vi "Create Cursor Plane.vi"(4 "Actual Range":T2, 5 "Cursor Plane":T3, 7 "Cursor Position":T1, 8 "error in (no error)":errorcluster, 11 "Cursor Object In":refnum<vi>) -> (0 "error out":errorcluster, 3 "Cursor Object Out":refnum<vi>)   [LabVIEW 2017, in "3D Plot.lvclass"]
uses:
  <vilib>/Math Plots/3D Math Plots/3D Plot/3D Plot/3D Plot.lvclass
  <vilib>/Math Plots/3D Math Plots/3D Plot/3D Plot/Typedef/Cursor Plane.ctl
  <vilib>/Math Plots/3D Math Plots/3D Plot/3D Plot/Typedef/Range Clusters.ctl
  <vilib>/picture/3D Picture Control/NI_3D Picture Control.lvlib
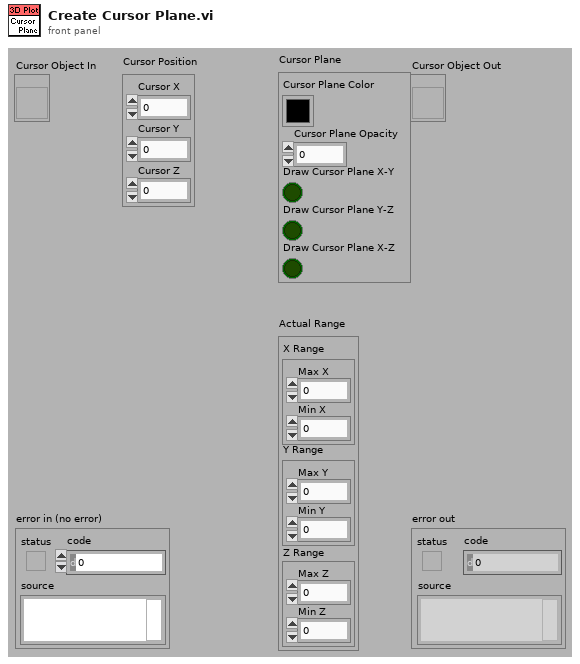
[diagram p1: front panel]
types:
  T1 = cluster{"Cursor X":sgl, "Cursor Y":sgl, "Cursor Z":sgl}
  T2 = typedef "3D Plot.lvclass/Range Clusters.ctl" = cluster{"X Range":cluster{"Max X":sgl, "Min X":sgl}, "Y Range":cluster{"Max Y":sgl, "Min Y":sgl}, "Z Range":cluster{"Max Z":sgl, "Min Z":sgl}}
  T3 = typedef "3D Plot.lvclass/Cursor Plane.ctl" = cluster{"Cursor Plane Color":u32, "Cursor Plane Opacity":sgl, "Draw Cursor Plane X-Z":bool, "Draw Cursor Plane Y-Z":bool, "Draw Cursor Plane X-Y":bool}
  T4 = enum16{"Normal Bin", "Opaque Bin", "Transparent Bin"}
  T5 = enum16{"Inherit Material", "Use entire Material", "Ignore Ambient", "Ignore Diffuse", "Ignore Specular", "Ignore Emission", "Ignore Ambient and Diffuse"}
  T6 = cluster{"X Range":cluster{"Max X":sgl, "Min X":sgl}, "Y Range":cluster{"Max Y":sgl, "Min Y":sgl}}
  T7 = cluster{"X Range":cluster{"Max X":sgl, "Min X":sgl}, "Z Range":cluster{"Max Z":sgl, "Min Z":sgl}}
  T8 = cluster{"Y Range":cluster{"Max Y":sgl, "Min Y":sgl}, "Z Range":cluster{"Max Z":sgl, "Min Z":sgl}}
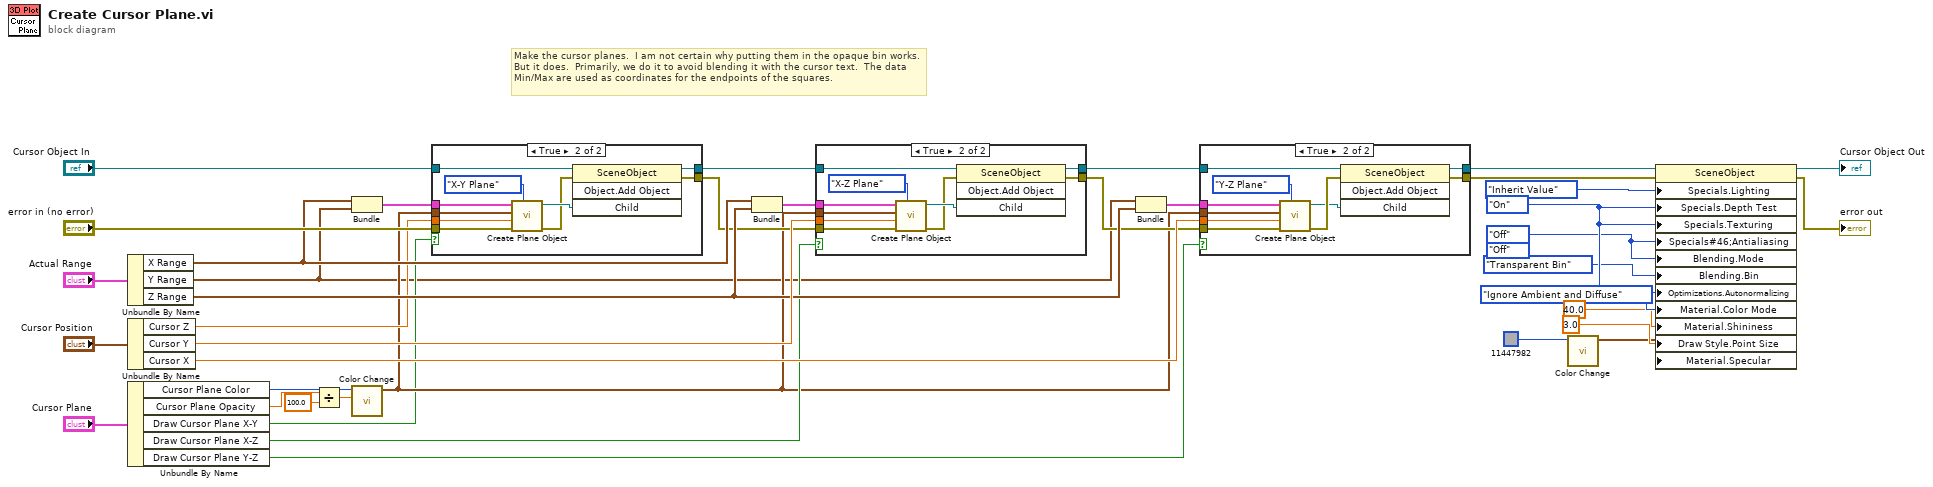
[diagram p0: block diagram]
diagram:
  (unwired) enum16{"Inherit Value", "Off", "On"}."Off" ("Blending:Mode")
  w6 = enum16{"Inherit Value", "Off", "On"}."On" ("Specials:Depth Test")
  w1 = enum16{"Inherit Value", "Off", "On"}."Off" ("Specials:Antialiasing")
  # "Make the cursor planes.  I am not certain why putting them in the opaque bin works.  But it does.  Primarily, we do it to avoid blending it with the cursor text.  The data Min/Max are used as coordinates for the endpoints of the squares."
  n1 = Unbundle By Name("Actual Range") -> ("X Range"=w27:cluster{"Max X":sgl, "Min X":sgl}, "Y Range"=w13:cluster{"Max Y":sgl, "Min Y":sgl}, "Z Range"=w26:cluster{"Max Z":sgl, "Min Z":sgl})
  n2 = Unbundle By Name("Cursor Position") -> ("Cursor Z"=w23:sgl, "Cursor Y"=w28:sgl, "Cursor X"=w24:sgl)
  n3 = Unbundle By Name("Cursor Plane") -> ("Cursor Plane Color"=w32:u32, "Cursor Plane Opacity"=w2:sgl, "Draw Cursor Plane X-Y"=w15:bool, "Draw Cursor Plane X-Z"=w22:bool, "Draw Cursor Plane Y-Z"=w21:bool)
  n4 = Divide(x=w2, y=sgl 100.0) -> (x/y=w17:sgl)
  n5 = Bundle("X Range"=w27, "Y Range"=w13) -> (w31:T6)  [unwired: 1 out]
  n6 = call <vilib>:"Color Change.vi"("Alpha"=w17, "Color"=w32) -> ("RGBA"=w16:cluster{"R":sgl, "G":sgl, "B":sgl, "A":sgl})  [unwired: 9 out]
  n7 = case shown="True" w15 {
    tunnel: w23 -> [_ w47]
    tunnel: w31 -> [_ w48]
    tunnel: w16 -> [_ w43]
    tunnel: "Cursor Object In" -> [w41 w51]
    tunnel: [w41 w49] -> w30
    tunnel: "error in (no error)" -> [w40 w46]
    tunnel: [w40 w50] -> w20
    frame False {
    }
    frame True {
      n8 = call <vilib>:"Create Plane Object.vi"("Plane"=enum16{"X-Y Plane", "Y-Z Plane", "X-Z Plane"}."X-Y Plane", "error in (no error)"=w46, "Offset"=w47, "RGBA"=w43, "Range Cluster"=w48) -> ("error out"=w44:errorcluster, "Cursor Plane Object"=w45:refnum<vi>)  [unwired: 1 in, 4 out]
      n9 = invoke class="SceneObject" method="Object.Add Object"(reference=w51, error in=w44, "Child"=w45) -> (reference out=w49:refnum<vi>, error out=w50:errorcluster)  [unwired: 1 in, 2 out]
    }
  }
  n10 = Bundle("X Range"=w27, "Z Range"=w26) -> (w14:T7)  [unwired: 1 out]
  n11 = case shown="True" w22 {
    tunnel: w28 -> [_ w60]
    tunnel: w14 -> [_ w59]
    tunnel: w16 -> [_ w55]
    tunnel: w30 -> [w53 w63]
    tunnel: [w53 w62] -> w29
    tunnel: w20 -> [w52 w56]
    tunnel: [w52 w61] -> w19
    frame False {
    }
    frame True {
      n12 = call <vilib>:"Create Plane Object.vi"("Plane"=enum16{"X-Y Plane", "Y-Z Plane", "X-Z Plane"}."X-Z Plane", "error in (no error)"=w56, "Offset"=w60, "RGBA"=w55, "Range Cluster"=w59) -> ("error out"=w57:errorcluster, "Cursor Plane Object"=w58:refnum<vi>)  [unwired: 1 in, 4 out]
      n13 = invoke class="SceneObject" method="Object.Add Object"(reference=w63, error in=w57, "Child"=w58) -> (reference out=w62:refnum<vi>, error out=w61:errorcluster)  [unwired: 1 in, 2 out]
    }
  }
  n14 = Bundle("Y Range"=w13, "Z Range"=w26) -> (w25:T8)  [unwired: 1 out]
  n15 = case shown="True" w21 {
    tunnel: w24 -> [_ w71]
    tunnel: w25 -> [_ w72]
    tunnel: w16 -> [_ w66]
    tunnel: w29 -> [w65 w75]
    tunnel: [w65 w74] -> w5
    tunnel: w19 -> [w64 w70]
    tunnel: [w64 w73] -> w4
    frame False {
    }
    frame True {
      n16 = call <vilib>:"Create Plane Object.vi"("Plane"=enum16{"X-Y Plane", "Y-Z Plane", "X-Z Plane"}."Y-Z Plane", "error in (no error)"=w70, "Offset"=w71, "RGBA"=w66, "Range Cluster"=w72) -> ("error out"=w69:errorcluster, "Cursor Plane Object"=w68:refnum<vi>)  [unwired: 1 in, 4 out]
      n17 = invoke class="SceneObject" method="Object.Add Object"(reference=w75, error in=w69, "Child"=w68) -> (reference out=w74:refnum<vi>, error out=w73:errorcluster)  [unwired: 1 in, 2 out]
    }
  }
  n18 = call <vilib>:"Color Change.vi"("Color"=u32 11447982) -> ("RGBA"=w7:cluster{"R":sgl, "G":sgl, "B":sgl, "A":sgl})  [unwired: 1 in, 9 out]
  n19 = property class="SceneObject"(reference=w5, error in=w4, "Specials.Lighting"=enum16{"Inherit Value", "Off", "On"}."Inherit Value" ("Specials:Lighting"), "Specials.Depth Test"=w6, "Specials.Texturing"=w6, "Specials#46;Antialiasing"=w1, "Blending.Mode"=w1, "Blending.Bin"=T4."Transparent Bin" ("Blending:Bin"), "Optimizations.Autonormalizing"=w6, "Material.Color Mode"=T5."Ignore Ambient and Diffuse" ("Material:Color Mode"), "Material.Shininess"=sgl 40.0 ("Material:Shininess"), "Draw Style.Point Size"=sgl 3.0 ("Draw Style:Point Size"), "Material.Specular"=w7) -> (reference out=→"Cursor Object Out":refnum<vi>, error out=→"error out":errorcluster)
